vi "string_to_int.vi"(8 "error in (no error)":errorcluster, 10 "Int (string)":string) -> (0 "error out":errorcluster, 2 "Int":i32)   [LabVIEW 2018]
doc: "Convert an IC6 response string representing an integer into a LabVIEW I32."
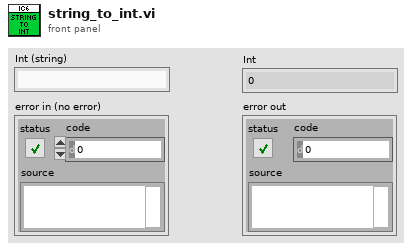
[diagram p1: front panel]
types:
  T1 = enum16{"big-endian, network order", "native, host order", "little-endian"}
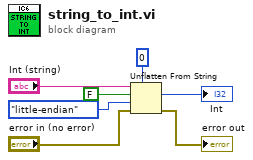
[diagram p0: block diagram]
diagram:
  n1 = Unflatten From String(type=0 ("offset (0)"), binary string="Int (string)", data includes array or string size? (T)=FALSE, byte order (0:big-endian, network order)=T1."little-endian", error in (no error)="error in (no error)") -> (value=→"Int":i32, error out=→"error out":errorcluster)  [unwired: 1 out]
